vi "DDS Generate RAM Data.vi"(8 "error in (no error)":errorcluster, 11 "DDS Channel":T3={"Power"=FALSE, "Channel Parameters"={"Ref Clock Rate [MHz]"=1000.0, "Full Scale Output\nPower [dBm]"=0.0}, "RAM Enable"=FALSE, "RAM Dest Type"=enum."Frequency", "RAM Default"={"Frequency [MHz]"=0.0, "Amplitude [dBm]"=0.0, "Phase Offset [rad]"=0.0}, "Array of DDS Profiles (8)"=[], "Description"=""} {"Array of DDS Profiles (8)"."Time Step (us)" min=0.0 max=262.14 step=0.004 format="%8.3g"; "Channel Parameters"."Ref Clock Rate [MHz]" min=0.0}) -> (0 "error out":errorcluster, 2 "RAM Profile Array":T1[](array[typedef]), 3 "RAM Word Array":u32[](array[numeric]))   [LabVIEW 2015, in "DDS.lvlib"]
uses:
  DDS.lvlib
  Controls/DDS Channel.ctl
  Controls/DDS Channel Parameters.ctl
  Controls/DDS RAM Destination.ctl
  Controls/DDS Profile Array.ctl
  Controls/DDS Profile.ctl
  Controls/DDS RAM Mode.ctl
  Controls/DDS RAM Timestep.ctl
  Controls/DDS RAM Profile.ctl
  <vilib>/gmath/NI_Gmath.lvlib
panel:
  out "Calculated Ramp":dbl[][](array[numeric])
  out "RAM Words by profile":u32[][](array[numeric])
  out "Static array empty?":bool[](array[boolean])
  out "Calculated Ramp":dbl[](array[numeric])
  # "f/f/A"
  # "Mag"
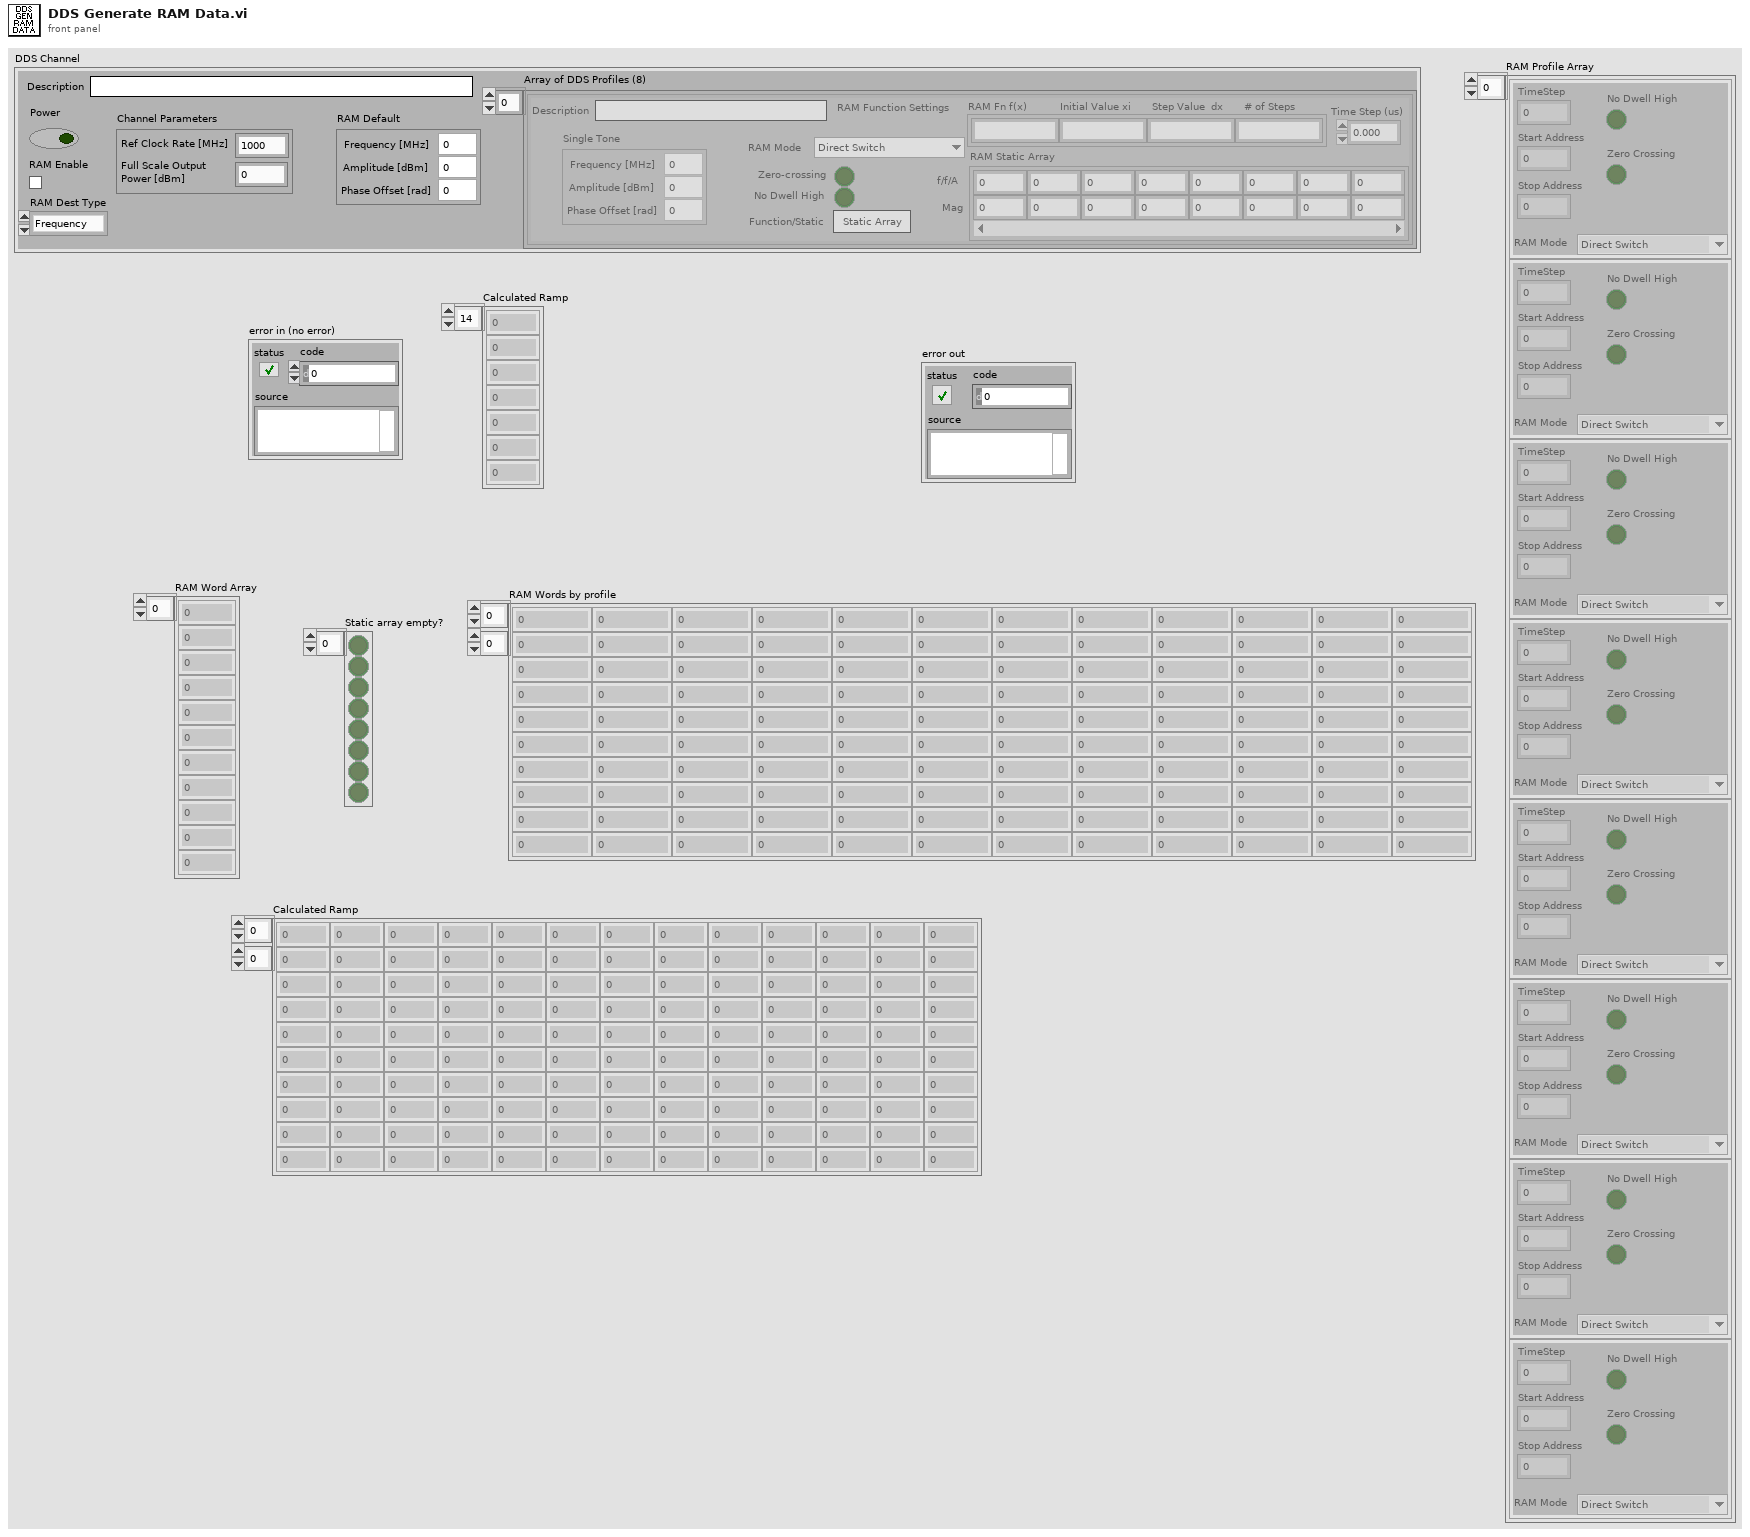
[diagram p1: front panel]
types:
  T1 = typedef "DDS.lvlib/DDS RAM Profile.ctl" = cluster{"TimeStep":u16, "Start Address":u16, "Stop Address":u16, "RAM Mode":T2, "No Dwell High":bool, "Zero Crossing":bool}
  T2 = typedef "DDS.lvlib/DDS RAM Mode.ctl" = enum16{"Direct Switch", "Ramp Up", "Bidirectional Ramp", "Continuous Bidirectional Ramp", "Continuous Recirculate", "Direct Switch 2", "Direct Switch 3", "Direct Switch 4"}
  T3 = typedef "DDS.lvlib/DDS Channel.ctl" = cluster{"Power":bool, "Channel Parameters":T4, "RAM Enable":bool, "RAM Dest Type":T5, "RAM Default":cluster{"Frequency [MHz]":dbl, "Amplitude [dBm]":dbl, "Phase Offset [rad]":dbl}, "Array of DDS Profiles (8)":T6, "Description":string}
  T4 = typedef "DDS.lvlib/DDS Channel Parameters.ctl" = cluster{"Ref Clock Rate [MHz]":dbl, "Full Scale Output\nPower [dBm]":dbl}
  T5 = typedef "DDS.lvlib/DDS RAM Destination.ctl" = enum16{"Frequency", "Phase", "Amplitude", "Polar"}
  T6 = typedef "DDS.lvlib/DDS Profile Array.ctl" = T7[]
  T7 = typedef "DDS.lvlib/DDS Profile.ctl" = cluster{"Single Tone":cluster{"Frequency [MHz]":dbl, "Amplitude [dBm]":dbl, "Phase Offset [rad]":dbl}, "RAM Mode ":T8, "Zero-crossing":bool, "No Dwell High":bool, "Function/Static":bool, "RAM Function Settings":string[], "RAM Static Array":dbl[][], "Description":string, "Time Step (us)":T9}
  T8 = typedef "DDS.lvlib/DDS RAM mode.ctl" = enum16{"Direct Switch", "Ramp Up", "Bidirectional Ramp", "Continuous Bidirectional Ramp", "Continuous Recirculate", "Direct Switch 2", "Direct Switch 3", "Direct Switch 4"}
  T9 = typedef "DDS.lvlib/DDS RAM Timestep.ctl" = dbl
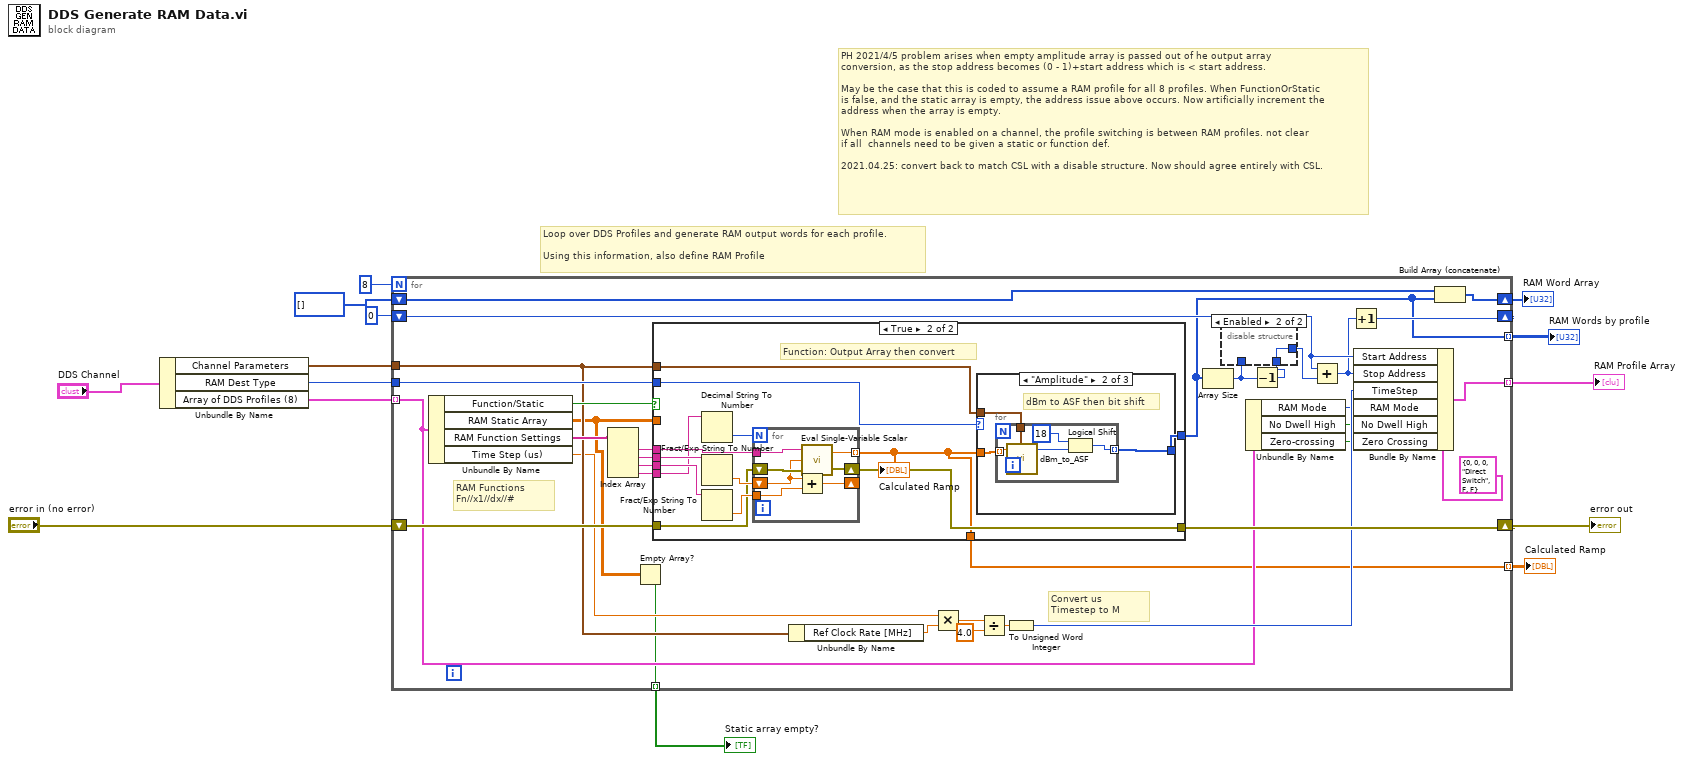
[diagram p0: block diagram]
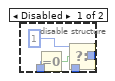
[diagram p2: hidden frame]
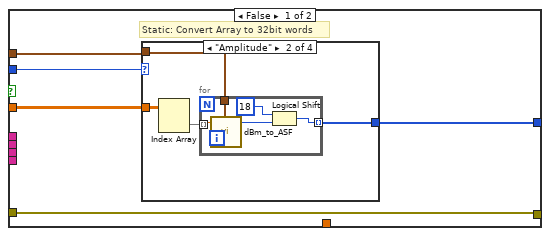
[diagram p3: hidden frame]
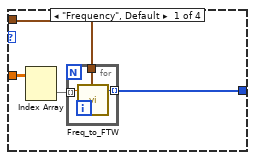
[diagram p4: hidden frame]
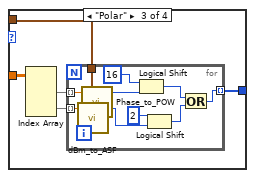
[diagram p5: hidden frame]
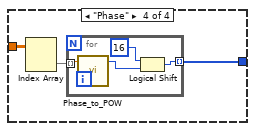
[diagram p6: hidden frame]
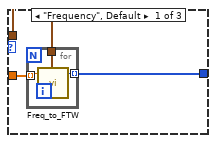
[diagram p7: hidden frame]
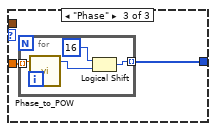
[diagram p8: hidden frame]
diagram:
  # "PH 2021/4/5 problem arises when empty amplitude array is passed out of he output array \nconversion, as the stop address becomes (0 - 1)+start address which is < start address. \n\nMay be the case that this is coded to assume a RAM profile for all 8 profiles. When FunctionOrStatic \nis false, and the static array is empty, the address issue above occurs. Now artificially increment the\naddress when the array is empty. \n\nWhen RAM mode is enabled on a channel, the profile switching is between RAM profiles. not clear\nif all  channels need to be given a static or function def.\n\n2021.04.25: convert back to match CSL with a disable structure. Now should agree entirely with CSL."
  # "Loop over DDS Profiles and generate RAM output words for each profile.\n\nUsing this information, also define RAM Profile"
  n1 = Unbundle By Name("DDS Channel") -> ("Channel Parameters"=w10:T4, "RAM Dest Type"=w11:T5, "Array of DDS Profiles (8)"=w12:T6)
  n2 = for {
    N: 8 -> [_]
    tunnel: w12 -> [w24] mode=indexing
    tunnel: w11 -> [w47]
    tunnel: w10 -> [w36]
    shift-right: [w46] -> w5
    shift-left: u32[] [] -> [w45]
    shift-right: [w39] -> w6
    shift-left: "error in (no error)" -> [w40]
    tunnel: [w32] -> w4 mode=indexing
    shift-right: [w29] -> _
    shift-left: u16 0 -> [w31]
    tunnel: [w20] -> w3 mode=indexing
    tunnel: [w16] -> w2 mode=indexing
    tunnel: [w15] -> w1 mode=indexing
    # "Convert us Timestep to M"
    # "RAM Functions\nFn//x1//dx//#"
    n3 = Unbundle By Name(w24) -> ("Function/Static"=w48:bool, "RAM Static Array"=w21:dbl[][], "RAM Function Settings"=w44:string[], "Time Step (us)"=w22:T9)
    n4 = Index Array(array=w44) -> (element #1=w43:string, element #2=w42:string, element #3=w41:string, element #4=w23:string)  [unwired: 4 in]
    n5 = Empty Array?(array=w21) -> (empty?=w20:bool)
    n6 = case shown="True" w48 {
      tunnel: w47 -> [w59 w107]
      tunnel: w21 -> [w55 _]
      tunnel: w36 -> [w58 w106]
      tunnel: [w57 w105] -> w16
      tunnel: w43 -> [_ w104]
      tunnel: w42 -> [_ w103]
      tunnel: w41 -> [_ w102]
      tunnel: w23 -> [_ w101]
      tunnel: w40 -> [w56 w100]
      tunnel: [w56 w99] -> w39
      tunnel: [_ w98] -> w15
      frame False {
        # "Static: Convert Array to 32bit words"
        n7 = case shown="\"Amplitude\"" w59 {
          tunnel: w55 -> [w63 w70 w80 w93]
          tunnel: w58 -> [w61 w68 w78 _]
          tunnel: [w60 w67 w77 w91] -> w57
          frame "Frequency", Default {
            n8 = Index Array(array=w63) -> (element=w62:dbl[])  [unwired: 2 in]
            n9 = for {
              tunnel: w62 -> [w66] mode=indexing
              tunnel: [w65] -> w60 mode=indexing
              tunnel: w61 -> [w64]
              n10 = call "Freq_to_FTW.vi"("Frequency (MHz)"=w66, "Channel Parameters"=w64) -> ("FTW (32bit)"=w65:u32)  [unwired: 25 in]
            }
          }
          frame "Amplitude" {
            n11 = Index Array(array=w70) -> (element=w69:dbl[])  [unwired: 2 in]
            n12 = for {
              tunnel: w69 -> [w75] mode=indexing
              tunnel: [w71] -> w67 mode=indexing
              tunnel: w68 -> [w74]
              n13 = call "dBm_to_ASF.vi"("Amplitude (dBm)"=w75, "Channel Parameters"=w74) -> ("ASF"=w73:u32)  [unwired: 25 in]
              n14 = Logical Shift(y=i8 18, x=w73) -> (x << y=w71:u32)
            }
          }
          frame "Polar" {
            n15 = Index Array(array=w80) -> (element #1=w79:dbl[], element #2=w76:dbl[])  [unwired: 4 in]
            n16 = for {
              tunnel: w79 -> [w85] mode=indexing
              tunnel: [w81] -> w77 mode=indexing
              tunnel: w78 -> [w90]
              tunnel: w76 -> [w88] mode=indexing
              n17 = call "dBm_to_ASF.vi"("Amplitude (dBm)"=w88, "Channel Parameters"=w90) -> ("ASF"=w87:u32)  [unwired: 25 in]
              n18 = call "Phase_to_POW.vi"("Phase (rad.)"=w85) -> ("POW"=w84:u32)  [unwired: 26 in]
              n19 = Logical Shift(y=i8 16, x=w84) -> (x << y=w82:u32)
              n20 = Logical Shift(y=i8 2, x=w87) -> (x << y=w83:u32)
              n21 = Or(x=w82, y=w83) -> (x .or. y?=w81:u32)
            }
          }
          frame "Phase" {
            n22 = Index Array(array=w93) -> (element=w92:dbl[])  [unwired: 2 in]
            n23 = for {
              tunnel: w92 -> [w97] mode=indexing
              tunnel: [w94] -> w91 mode=indexing
              n24 = call "Phase_to_POW.vi"("Phase (rad.)"=w97) -> ("POW"=w96:u32)  [unwired: 26 in]
              n25 = Logical Shift(y=i8 16, x=w96) -> (x << y=w94:u32)
            }
          }
        }
      }
      frame True {
        # "Function: Output Array then convert"
        n26 = Decimal String To Number(string=w101) -> (number=w108:i32)  [unwired: 2 in, 1 out]
        n27 = Fract/Exp String To Number(string=w103) -> (number=w110:dbl)  [unwired: 3 in, 1 out]
        n28 = Fract/Exp String To Number(string=w102) -> (number=w109:dbl)  [unwired: 3 in, 1 out]
        n29 = for {
          N: w108 -> [_]
          tunnel: w104 -> [w137]
          tunnel: [w136] -> w98 mode=indexing
          shift-right: [w135] -> _
          shift-left: w110 -> [w132]
          tunnel: w109 -> [w131]
          shift-right: [w134] -> w99
          shift-left: w100 -> [w133]
          n30 = Add(x=w132, y=w131) -> (x+y=w135:dbl)
          n31 = call <vilib>:"Eval Single-Variable Scalar.vi"("error in (no error)"=w133, "x value"=w132, "formula"=w137) -> ("error out"=w134:errorcluster, "y value"=w136:dbl)
        }
        "Calculated Ramp" <- w98
        n32 = case shown="\"Amplitude\"" w107 {
          tunnel: w106 -> [w113 w119 _]
          tunnel: [w112 w118 w126] -> w105
          tunnel: w98 -> [w111 w117 w125]
          frame "Frequency", Default {
            n33 = for {
              tunnel: w111 -> [w116] mode=indexing
              tunnel: [w115] -> w112 mode=indexing
              tunnel: w113 -> [w114]
              n34 = call "Freq_to_FTW.vi"("Frequency (MHz)"=w116, "Channel Parameters"=w114) -> ("FTW (32bit)"=w115:u32)  [unwired: 25 in]
            }
          }
          frame "Amplitude" {
            # "dBm to ASF then bit shift"
            n35 = for {
              tunnel: w117 -> [w124] mode=indexing
              tunnel: [w120] -> w118 mode=indexing
              tunnel: w119 -> [w123]
              n36 = call "dBm_to_ASF.vi"("Amplitude (dBm)"=w124, "Channel Parameters"=w123) -> ("ASF"=w122:u32)  [unwired: 25 in]
              n37 = Logical Shift(y=i8 18, x=w122) -> (x << y=w120:u32)
            }
          }
          frame "Phase" {
            n38 = for {
              tunnel: w125 -> [w130] mode=indexing
              tunnel: [w127] -> w126 mode=indexing
              n39 = call "Phase_to_POW.vi"("Phase (rad.)"=w130) -> ("POW"=w129:u32)  [unwired: 26 in]
              n40 = Logical Shift(y=i8 16, x=w129) -> (x << y=w127:u32)
            }
          }
        }
      }
    }
    n41 = Unbundle By Name(w36) -> ("Ref Clock Rate [MHz]"=w35:dbl)
    n42 = Multiply(x=w22, y=w35) -> (x*y=w38:T9)
    n43 = Divide(x=w38, y=4.0) -> (x/y=w34:T9)
    n44 = To Unsigned Word Integer(number=w34) -> (unsigned 16bit integer=w28:u16)
    n45 = Array Size(array=w16) -> (size(s)=w19:i32)
    n46 = Unbundle By Name(w24) -> ("RAM Mode"=w27:T8, "No Dwell High"=w26:bool, "Zero-crossing"=w25:bool)
    n47 = Decrement(x=w19) -> (x-1=w18:i32)
    n48 = disable-structure shown="Enabled" {
      disable-tunnel: w19 -> [w53 _]
      disable-tunnel: w18 -> [w52 w54]
      disable-tunnel: [w49 w54] -> w17
      frame Disabled {
        n49 = Equal To 0?(x=w53) -> (x = 0?=w51:bool)
        n50 = Select(t=1, s=w51, f=w52) -> (s? t:f=w49:i32)
      }
      frame Enabled {
      }
    }
    n51 = Add(x=w31, y=w17) -> (x+y=w30:i32)
    n52 = Increment(x=w30) -> (x+1=w29:i32)
    n53 = Bundle By Name(cluster=T1 {"TimeStep"=0, "Start Address"=0, "Stop Address"=0, "RAM Mode"=enum."Direct Switch", "No Dwell High"=FALSE, "Zero Crossing"=FALSE} ("Cluster"), "Start Address"=w31, "Stop Address"=w30, "TimeStep"=w28, "RAM Mode"=w27, "No Dwell High"=w26, "Zero Crossing"=w25) -> (w32:T1)
    n54 = Build Array (concatenate)(w45, w16) -> (w46:u32[])
  }
  "error out" <- w6
  "RAM Word Array" <- w5
  "RAM Profile Array" <- w4
  "Static array empty?" <- w3
  "RAM Words by profile" <- w2
  "Calculated Ramp" <- w1
